vi "Begin.vi"(8 "error in":errorcluster) -> (0 "error out":errorcluster)   [LabVIEW 2018]
doc: "Called before other user functions, this VI is expected to open initial I/O refnums, load in file data, and do all program initialization. Notice that the <B>error out</B> terminal is simply used for data flow. Wiring it to other structures or subVIs ensures that this VI runs first."
uses:
  <vilib>/Rock Robotics/WPI/ThirdParty/Phoenix-LabVIEW/Motor Controller/Controls/CTRE_Phoenix_MotorControl_EnhancedMotorControllerConfigurables.ctl
  <vilib>/Rock Robotics/WPI/ThirdParty/Phoenix-LabVIEW/Motor Controller/Controls/CTRE_Phoenix_MotorControl_BaseConfigurables.ctl
  <vilib>/Rock Robotics/WPI/ThirdParty/Phoenix-LabVIEW/Motor Controller/Controls/CTRE_Phoenix_MotorControl_VelocityMeasurementPeriod.ctl
  <vilib>/Rock Robotics/WPI/ThirdParty/Phoenix-LabVIEW/Motor Controller/Controls/CTRE_Phoenix_MotorControl_SlotStructure.ctl
  <vilib>/Rock Robotics/WPI/ThirdParty/Phoenix-LabVIEW/Motor Controller/Controls/CTRE_Phoenix_MotorControl_FilterStruct.ctl
  <vilib>/Rock Robotics/WPI/ThirdParty/Phoenix-LabVIEW/Motor Controller/Controls/CTRE_Phoenix_MotorControl_RemoteSourceType.ctl
  <vilib>/Rock Robotics/WPI/ThirdParty/Phoenix-LabVIEW/Controls/CTRE_Phoenix_CustomParamConfiguration.ctl
  <vilib>/Rock Robotics/WPI/ThirdParty/Phoenix-LabVIEW/Motor Controller/Controls/CTRE_Phoenix_MotorControl_FeedbackDevice.ctl
  <vilib>/Rock Robotics/WPI/ThirdParty/Phoenix-LabVIEW/Motor Controller/Controls/CTRE_Phoenix_MotorControl_SensorTermFeedbackDevice_Enhanced.ctl
  <vilib>/Rock Robotics/WPI/ThirdParty/Phoenix-LabVIEW/Motor Controller/Controls/CTRE_Phoenix_MotorControl_LimitSwitchNormal.ctl
  <vilib>/Rock Robotics/WPI/ThirdParty/Phoenix-LabVIEW/Motor Controller/Controls/CTRE_Phoenix_MotorControl_LimitSwitchSource_Local.ctl
  <vilib>/Rock Robotics/WPI/ThirdParty/Phoenix-LabVIEW/Motor Controller/Controls/CTRE_Phoenix_MotorControl_MotorControllerConfigurables.ctl
  <vilib>/Rock Robotics/WPI/ThirdParty/Phoenix-LabVIEW/Motor Controller/Controls/CTRE_Phoenix_MotorControl_RemoteFeedbackDevice.ctl
  <vilib>/Rock Robotics/WPI/ThirdParty/Phoenix-LabVIEW/Motor Controller/Controls/CTRE_Phoenix_MotorControl_SensorTermFeedbackDevice.ctl
  <vilib>/Rock Robotics/WPI/ThirdParty/Phoenix-LabVIEW/Motor Controller/Controls/CTRE_Phoenix_MotorControl_LimitSwitchSource.ctl
  <vilib>/Rock Robotics/WPI/DriverStation/WPI_DriverStationRobotMode2.ctl
  <vilib>/Rock Robotics/WPI/Joystick/WPI_JoystickDeviceEnum.ctl
  <vilib>/Rock Robotics/WPI/Solenoid/WPI_SolenoidChannel.ctl
  <vilib>/Rock Robotics/SystemInterfaces/AI/FPGA_AIChannel.ctl
  <vilib>/Rock Robotics/WPI/ThirdParty/Phoenix-LabVIEW/Motor Controller/Controls/CTRE_Phoenix_MotorControl_NeutralMode.ctl
  <vilib>/Rock Robotics/WPI/Accelerometer/WPI_AccelerometerRange.ctl
  <vilib>/Rock Robotics/WPI/ThirdParty/REV Robotics/SPARK MAX/Typedef/Spark MAX Idle Mode.ctl
  <vilib>/Rock Robotics/SystemInterfaces/DIO/FPGA_DIOPWMChannel.ctl
  Robot Global Data.vi
  RefNums_DriverStation.vi
  <vilib>/Rock Robotics/Network Tables/NT Write String Array.vi
  <vilib>/Rock Robotics/WPI/Solenoid/WPI_SolenoidOpenDouble.vi
  RefNums_Actuators.vi
  <vilib>/Rock Robotics/WPI/Utilities/WPI_GetSetVariantRefNum.vi
  RefNums_Sensors.vi
  <vilib>/Rock Robotics/WPI/Accelerometer/InternalAccelerometer/WPI_AccelerometerInternalOpen.vi
  <vilib>/Rock Robotics/WPI/Solenoid/WPI_SolenoidOpenSingle.vi
  <vilib>/Rock Robotics/WPI/SafetyOutput/WPI_SafetyOutputConfigMenu.ctl
  <vilib>/Rock Robotics/WPI/RobotDrive/WPI_RobotDriveOpen4MotorWithExistingMotors.vi
panel:
  in  "Victor Enhanced Control":T1={"Base Configurables"={"openLoopRamp"=0.0, "closedLoopRamp"=0.0, "peakOutputForward"=1.0, "peakOutputReverse"=-1.0, "nominalOutputForward"=0.0, "nominalOutputReverse"=0.0, "neutralDeadband"=0.04, "voltageCompSaturation"=0.0, "voltageMeasurementFilter"=32, "velocityMeasurementPeriod"=100, "velocityMeasurementWindow"=64, "forwardSoftLimitThreshold"=0, "reverseSoftLimitThreshold"=0, "forwardSoftLimitEnable"=FALSE, "reverseSoftLimitEnable"=FALSE, "slot0"={"P"=0.0, "I"=0.0, "D"=0.0, "F"=0.0, "integralZone"=0.0, "allowableClosedLoopError"=0, "maxIntegralAccumulator"=0.0, "closedLoopPeakOutput"=1.0, "closedLoopPeriod"=1}, "slot1"={"P"=0.0, "I"=0.0, "D"=0.0, "F"=0.0, "integralZone"=0.0, "allowableClosedLoopError"=0, "maxIntegralAccumulator"=0.0, "closedLoopPeakOutput"=1.0, "closedLoopPeriod"=1}, "slot2"={"P"=0.0, "I"=0.0, "D"=0.0, "F"=0.0, "integralZone"=0.0, "allowableClosedLoopError"=0, "maxIntegralAccumulator"=0.0, "closedLoopPeakOutput"=1.0, "closedLoopPeriod"=1}, "slot3"={"P"=0.0, "I"=0.0, "D"=0.0, "F"=0.0, "integralZone"=0.0, "allowableClosedLoopError"=0, "maxIntegralAccumulator"=0.0, "closedLoopPeakOutput"=1.0, "closedLoopPeriod"=1}, "auxPIDPolarity"=FALSE, "remoteFilter0"={"remoteSensorDeviceID"=0, "remoteSensorSource"=enum."Off"}, "remoteFilter1"={"remoteSensorDeviceID"=0, "remoteSensorSource"=enum."Off"}, "motionCruiseVelocity"=0, "motionAcceleration"=0, "motionProfileTrajectoryPeriod"=0, "feedbackNotContinuous"=FALSE, "remoteSensorClosedLoopDisableNeutralOnLOS"=FALSE, "clearPositionOnLimitF"=FALSE, "clearPositionOnLimitR"=FALSE, "clearPositionOnQuadIdx"=FALSE, "limitSwitchDisableNeutralOnLOS"=FALSE, "softLimitDisableNeutralOnLOS"=FALSE, "pulseWidthPeriod_EdgesPerRot"=1, "pulseWidthPeriod_FilterWindowSz"=1, "customParam"={"customParam0"=0, "customParam1"=0}, "trajectoryInterpolationEnable"=TRUE}, "primaryPID"={"selectedFeedbackCoefficient"=1.0, "selectedFeedbackSensor"=11}, "auxiliaryPID"={"selectedFeedbackCoefficient"=1.0, "selectedFeedbackSensor"=11}, "sum 0 term"=11, "sum 1 term"=11, "diff 0 term "=11, "diff 1 term"=11, "forwardLimitSwitchDeviceID"=0, "reverseLimitSwitchDeviceID"=0, "forwardLimitSwitchNormal"=enum."Normally Open", "reverseLimitSwitchNormal"=enum."Normally Open", "forwardLimitSwitchSource"=3, "reverseLimitSwitchSource"=3} {"diff 1 term" items=["Remote Source 0"=11, "Remote Source 1"=12, "Software Emulated"=15]; "diff 0 term" items=["Remote Source 0"=11, "Remote Source 1"=12, "Software Emulated"=15]; "sum 1 term" items=["Remote Source 0"=11, "Remote Source 1"=12, "Software Emulated"=15]; "sum 0 term" items=["Remote Source 0"=11, "Remote Source 1"=12, "Software Emulated"=15]; "reverseLimitSwitchSource" items=["Remote Talon SRX"=1, "Remote CANifier"=2, "Deactivated"=3]; "forwardLimitSwitchSource" items=["Remote Talon SRX"=1, "Remote CANifier"=2, "Deactivated"=3]; "auxiliaryPID"."selectedFeedbackSensor" items=["Sensor Sum (S0 + S1)"=9, "Sensor Difference (D0 - D1)"=10, "Remote Source 0"=11, "Remote Source 1"=12, "Software Emulated"=15]; "primaryPID"."selectedFeedbackSensor" items=["Sensor Sum (S0 + S1)"=9, "Sensor Difference (D0 - D1)"=10, "Remote Source 0"=11, "Remote Source 1"=12, "Software Emulated"=15]; "Base Configurables"."velocityMeasurementPeriod" items=["Period_1ms"=1, "Period_2ms"=2, "Period_5ms"=5, "Period_10ms"=10, "Period_20ms"=20, "Period_25ms"=25, "Period_50ms"=50, "Period_100ms"=100]}
  in  "Talon Enhanced Config":T12={"Base Configurables"={"openLoopRamp"=0.0, "closedLoopRamp"=0.0, "peakOutputForward"=1.0, "peakOutputReverse"=-1.0, "nominalOutputForward"=0.0, "nominalOutputReverse"=0.0, "neutralDeadband"=0.04, "voltageCompSaturation"=0.0, "voltageMeasurementFilter"=32, "velocityMeasurementPeriod"=100, "velocityMeasurementWindow"=64, "forwardSoftLimitThreshold"=0, "reverseSoftLimitThreshold"=0, "forwardSoftLimitEnable"=FALSE, "reverseSoftLimitEnable"=FALSE, "slot0"={"P"=0.0, "I"=0.0, "D"=0.0, "F"=0.0, "integralZone"=0.0, "allowableClosedLoopError"=0, "maxIntegralAccumulator"=0.0, "closedLoopPeakOutput"=1.0, "closedLoopPeriod"=1}, "slot1"={"P"=0.0, "I"=0.0, "D"=0.0, "F"=0.0, "integralZone"=0.0, "allowableClosedLoopError"=0, "maxIntegralAccumulator"=0.0, "closedLoopPeakOutput"=1.0, "closedLoopPeriod"=1}, "slot2"={"P"=0.0, "I"=0.0, "D"=0.0, "F"=0.0, "integralZone"=0.0, "allowableClosedLoopError"=0, "maxIntegralAccumulator"=0.0, "closedLoopPeakOutput"=1.0, "closedLoopPeriod"=1}, "slot3"={"P"=0.0, "I"=0.0, "D"=0.0, "F"=0.0, "integralZone"=0.0, "allowableClosedLoopError"=0, "maxIntegralAccumulator"=0.0, "closedLoopPeakOutput"=1.0, "closedLoopPeriod"=1}, "auxPIDPolarity"=FALSE, "remoteFilter0"={"remoteSensorDeviceID"=0, "remoteSensorSource"=enum."Off"}, "remoteFilter1"={"remoteSensorDeviceID"=0, "remoteSensorSource"=enum."Off"}, "motionCruiseVelocity"=0, "motionAcceleration"=0, "motionProfileTrajectoryPeriod"=0, "feedbackNotContinuous"=FALSE, "remoteSensorClosedLoopDisableNeutralOnLOS"=FALSE, "clearPositionOnLimitF"=FALSE, "clearPositionOnLimitR"=FALSE, "clearPositionOnQuadIdx"=FALSE, "limitSwitchDisableNeutralOnLOS"=FALSE, "softLimitDisableNeutralOnLOS"=FALSE, "pulseWidthPeriod_EdgesPerRot"=1, "pulseWidthPeriod_FilterWindowSz"=1, "customParam"={"customParam0"=0, "customParam1"=0}, "trajectoryInterpolationEnable"=TRUE}, "primaryPID"={"selectedFeedbackCoefficient"=1.0, "selectedFeedbackSensor"=0}, "auxiliaryPID"={"selectedFeedbackCoefficient"=1.0, "selectedFeedbackSensor"=0}, "sum0Term"=0, "sum1Term"=0, "diff0Term"=0, "diff1Term"=0, "forwardLimitSwitchNormal"=enum."Normally Open", "reverseLimitSwitchNormal"=enum."Normally Open", "forwardLimitSwitchDeviceID"=0, "reverseLimitSwitchDeviceID"=0, "forwardLimitSwitchSource"=enum."Feedback Connector", "reverseLimitSwitchSource"=enum."Feedback Connector", "peakCurrentLimit"=1, "peakCurrentDuration"=1, "continuousCurrentLimit"=1} {"diff1Term" items=["QuadEncoder"=0, "Analog"=2, "Tachometer"=4, "Pulse Width Encoded Position"=8, "Remote Source 0"=11, "Remote Source 1"=12, "Software Emulated"=15]; "diff0Term" items=["QuadEncoder"=0, "Analog"=2, "Tachometer"=4, "Pulse Width Encoded Position"=8, "Remote Source 0"=11, "Remote Source 1"=12, "Software Emulated"=15]; "sum1Term" items=["QuadEncoder"=0, "Analog"=2, "Tachometer"=4, "Pulse Width Encoded Position"=8, "Remote Source 0"=11, "Remote Source 1"=12, "Software Emulated"=15]; "sum0Term" items=["QuadEncoder"=0, "Analog"=2, "Tachometer"=4, "Pulse Width Encoded Position"=8, "Remote Source 0"=11, "Remote Source 1"=12, "Software Emulated"=15]; "auxiliaryPID"."selectedFeedbackSensor" items=["QuadEncoder"=0, "Analog"=2, "Tachometer"=4, "Pulse Width Encoded Position"=8, "Sensor Sum (S0 + S1)"=9, "Sensor Difference (D0 - D1)"=10, "Remote Source 0"=11, "Remote Source 1"=12, "Software Emulated"=15]; "primaryPID"."selectedFeedbackSensor" items=["QuadEncoder"=0, "Analog"=2, "Tachometer"=4, "Pulse Width Encoded Position"=8, "Sensor Sum (S0 + S1)"=9, "Sensor Difference (D0 - D1)"=10, "Remote Source 0"=11, "Remote Source 1"=12, "Software Emulated"=15]; "Base Configurables"."velocityMeasurementPeriod" items=["Period_1ms"=1, "Period_2ms"=2, "Period_5ms"=5, "Period_10ms"=10, "Period_20ms"=20, "Period_25ms"=25, "Period_50ms"=50, "Period_100ms"=100]}
  # "Sum and Diff terms are ways to select more than one sensor as a feedback device. \n Sum 0 is the first feedback device to be used for the Sum term, \n Sum 1 is the feedback device to be added to Sum 0 for the Sum term\n Diff 0 and Diff 1 work in a similar manner"
  # "These are only applicable\nif using a remote limit switch.\n\nLocal limit switches/no limit\nswitches do not use this"
  # "False: Primary Output = PID[0] + PID[1]  ---  Auxiliary Output = PID[0] - PID[1]\nTrue:  Primary Output = PID[0] - PID[1] --- Auxiliary Output = PID[0] + PID[1]"
  # "Enable the motion profile executor to perform linear interpolation between profile points.  Defaults to True."
  # "Sum and Diff terms are ways to select more than one sensor as a feedback device. \n Sum 0 is the first feedback device to be used for the Sum term.\n Sum 1 is the feedback device to be added to Sum 0 for the Sum term.\n Diff 0 and Diff 1 work in a similar manner."
  # "These are only applicable\nif using a remote limit switch.\n\nLocal limit switches/no limit\nswitches do not use this."
  # "Current is below Continuous threshold AND\n\n(Requested output is weaker** than applied motor\noutput OR is in the opposite direction).\n/\nMotor output is set to requested output."
  # "Current is above Peak* Threshold for Peak Duration.\n/\nReduce motor output (towards neutral)."
  # "Current is below Continuous threshold.\n/\nRamp motor output towards requested output."
  # "Current is above Continuous threshold.\n/\nReduce motor output (towards neutral)."
  # "Current Limiting is NOT enabled\nby default.\nCall this VI to enable."
  # "*If the configured Peak Threshold is less than the Continuous Threshold, the applied Peak Threshold is set equal to the Configured Continuous Threshold in firmware.\n** Both requested output and applied motor output are in the same direction, and requested output is closer to neutral."
  # "False: Primary Output = PID[0] + PID[1]  ---  Auxiliary Output = PID[0] - PID[1]\nTrue:  Primary Output = PID[0] - PID[1] --- Auxiliary Output = PID[0] + PID[1]"
  # "Enable the motion profile executor to perform linear interpolation between profile points.  Defaults to True."
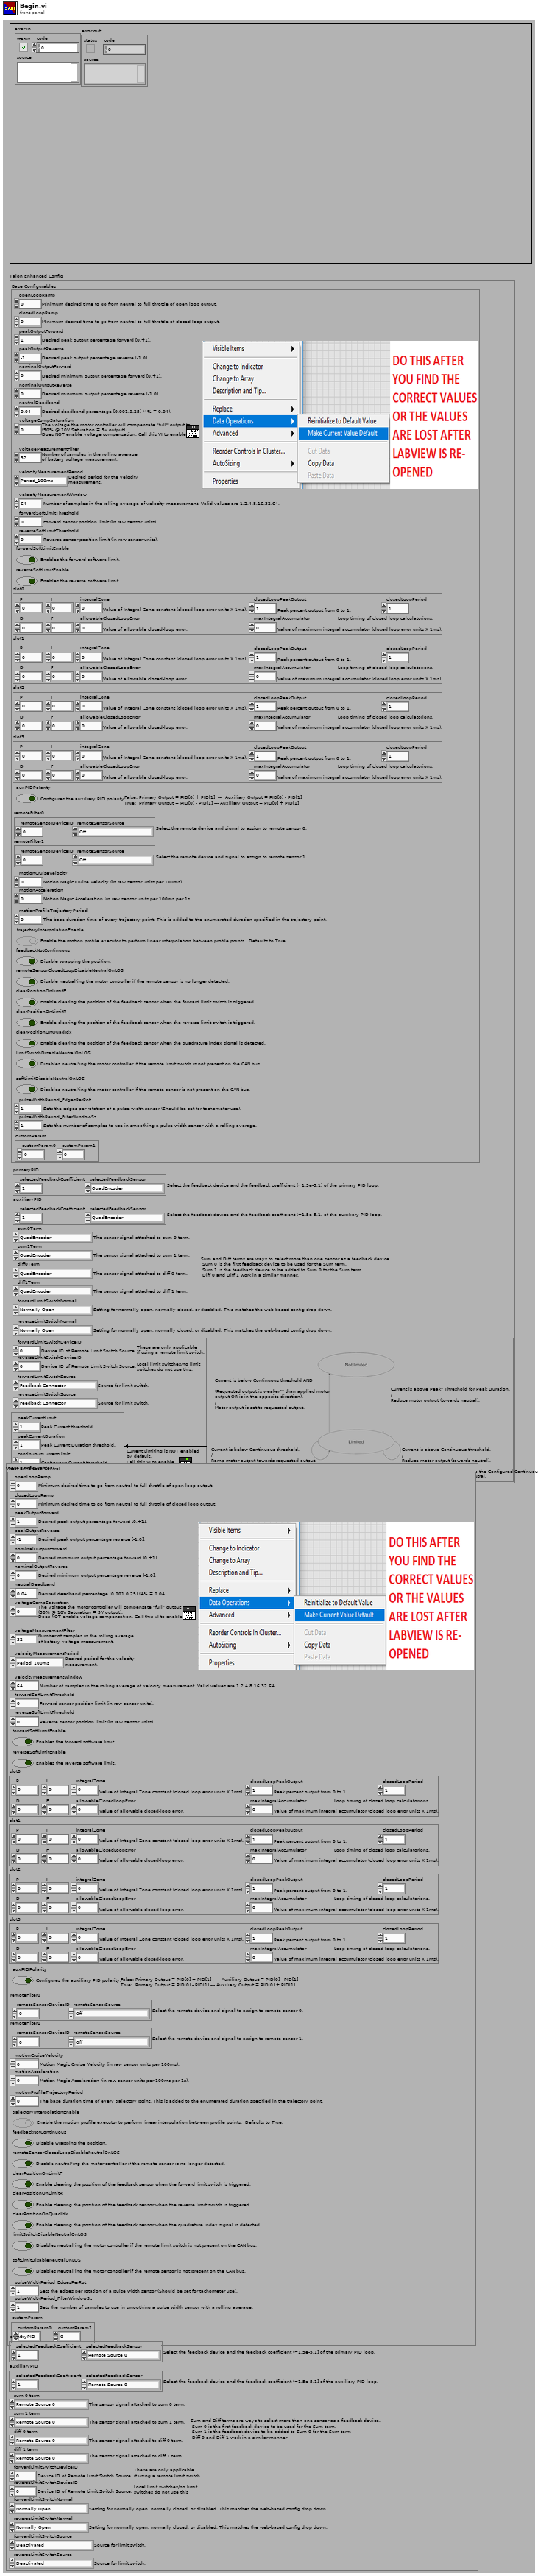
[diagram p1: front panel]
types:
  T1 = typedef "CTRE_Phoenix_MotorControl_MotorControllerConfigurables.ctl" = cluster{"Base Configurables":T2, "primaryPID":cluster{"selectedFeedbackCoefficient":dbl, "selectedFeedbackSensor":T8}, "auxiliaryPID":cluster{"selectedFeedbackCoefficient":dbl, "selectedFeedbackSensor":T8}, "sum 0 term":T9, "sum 1 term":T9, "diff 0 term ":T9, "diff 1 term":T9, "forwardLimitSwitchDeviceID":i32, "reverseLimitSwitchDeviceID":i32, "forwardLimitSwitchNormal":T10, "reverseLimitSwitchNormal":T10, "forwardLimitSwitchSource":T11, "reverseLimitSwitchSource":T11}
  T2 = typedef "CTRE_Phoenix_MotorControl_BaseConfigurables.ctl" = cluster{"openLoopRamp":dbl, "closedLoopRamp":dbl, "peakOutputForward":dbl, "peakOutputReverse":dbl, "nominalOutputForward":dbl, "nominalOutputReverse":dbl, "neutralDeadband":dbl, "voltageCompSaturation":dbl, "voltageMeasurementFilter":i32, "velocityMeasurementPeriod":T3, "velocityMeasurementWindow":i32, "forwardSoftLimitThreshold":i32, "reverseSoftLimitThreshold":i32, "forwardSoftLimitEnable":bool, "reverseSoftLimitEnable":bool, "slot0":T4, "slot1":T4, "slot2":T4, "slot3":T4, "auxPIDPolarity":bool, "remoteFilter0":T5, "remoteFilter1":T5, "motionCruiseVelocity":i32, "motionAcceleration":i32, "motionProfileTrajectoryPeriod":i32, "feedbackNotContinuous":bool, "remoteSensorClosedLoopDisableNeutralOnLOS":bool, "clearPositionOnLimitF":bool, "clearPositionOnLimitR":bool, "clearPositionOnQuadIdx":bool, "limitSwitchDisableNeutralOnLOS":bool, "softLimitDisableNeutralOnLOS":bool, "pulseWidthPeriod_EdgesPerRot":i32, "pulseWidthPeriod_FilterWindowSz":i32, "customParam":T7, "trajectoryInterpolationEnable":bool}
  T3 = typedef "CTRE_Phoenix_MotorControl_VelocityMeasurementPeriod.ctl" = u16
  T4 = typedef "CTRE_Phoenix_MotorControl_SlotStructure.ctl" = cluster{"P":dbl, "I":dbl, "D":dbl, "F":dbl, "integralZone":dbl, "allowableClosedLoopError":i32, "maxIntegralAccumulator":dbl, "closedLoopPeakOutput":dbl, "closedLoopPeriod":i32}
  T5 = typedef "CTRE_Phoenix_MotorControl_FilterStruct.ctl" = cluster{"remoteSensorDeviceID":u8, "remoteSensorSource":T6}
  T6 = typedef "CTRE_Phoenix_MotorControl_RemoteSourceType.ctl" = enum16{"Off", "Talon SRX Selected Sensor", "Pigeon IMU Yaw", "Pigeon IMU Pitch", "Pigeon IMU Roll", "CANifier Quadrature", "CANifier PWM Input 0", "CANifier PWM Input 1", "CANifier PWM Input 2", "CANifier PWM Input 3", "Gadgeteer Pigeon Yaw", "Gadgeteer Pigeon Pitch", "Gadgeteer Pigeon Roll"}
  T7 = typedef "CTRE_Phoenix_CustomParamConfiguration.ctl" = cluster{"customParam0":i32, "customParam1":i32}
  T8 = typedef "CTRE_Phoenix_MotorControl_RemoteFeedbackDevice.ctl" = i8
  T9 = typedef "CTRE_Phoenix_MotorControl_SensorTermFeedbackDevice.ctl" = i8
  T10 = typedef "CTRE_Phoenix_MotorControl_LimitSwitchNormal.ctl" = enum16{"Normally Open", "Normally Closed", "Disabled"}
  T11 = typedef "CTRE_Phoenix_MotorControl_LimitSwitchSource.ctl" = u16
  T12 = typedef "CTRE_Phoenix_MotorControl_EnhancedMotorControllerConfigurables.ctl" = cluster{"Base Configurables":T2, "primaryPID":cluster{"selectedFeedbackCoefficient":dbl, "selectedFeedbackSensor":T13}, "auxiliaryPID":cluster{"selectedFeedbackCoefficient":dbl, "selectedFeedbackSensor":T13}, "sum0Term":T14, "sum1Term":T14, "diff0Term":T14, "diff1Term":T14, "forwardLimitSwitchNormal":T10, "reverseLimitSwitchNormal":T10, "forwardLimitSwitchDeviceID":i32, "reverseLimitSwitchDeviceID":i32, "forwardLimitSwitchSource":T15, "reverseLimitSwitchSource":T15, "peakCurrentLimit":i32, "peakCurrentDuration":i32, "continuousCurrentLimit":i32}
  T13 = typedef "CTRE_Phoenix_MotorControl_FeedbackDevice.ctl" = i8
  T14 = typedef "CTRE_Phoenix_MotorControl_SensorTermFeedbackDevice_Enhanced.ctl" = i8
  T15 = typedef "CTRE_Phoenix_MotorControl_LimitSwitchSource_Local.ctl" = enum16{"Feedback Connector", "Remote Talon SRX", "Remote CANifier", "Deactivated"}
  T16 = typedef "FPGA_DIOPWMChannel.ctl" = enum8{"PWM 0", "PWM 1", "PWM 2", "PWM 3", "PWM 4", "PWM 5", "PWM 6", "PWM 7", "PWM 8", "PWM 9", "PWM MXP 0", "PWM MXP 1", "PWM MXP 2", "PWM MXP 3", "PWM MXP 4", "PWM MXP 5", "PWM MXP 6", "PWM MXP 7", "PWM MXP 8", "PWM MXP 9", "Invalid"}
  T17 = typedef "Spark MAX Idle Mode.ctl" = enum16{"Coast", "Brake"}
  T18 = typedef "WPI_SolenoidChannel.ctl" = enum8{"Solenoid 0", "Solenoid 1", "Solenoid 2", "Solenoid 3", "Solenoid 4", "Solenoid 5", "Solenoid 6", "Solenoid 7", "Invalid"}
  T19 = typedef "WPI_AccelerometerRange.ctl" = enum16{"+/- 2 g", "+/- 4 g", "+/- 8 g"}
  T20 = typedef "WPI_JoystickDeviceEnum.ctl" = enum16{"USB 0", "USB 1", "USB 2", "USB 3", "USB 4", "USB 5"}
  T21 = typedef "CTRE_Phoenix_MotorControl_NeutralMode.ctl" = enum8{"EEPROMSetting", "Override to Coast", "Override to Brake"}
  T22 = typedef "FPGA_AIChannel.ctl" = enum8{"AI 0", "AI 1", "AI 2", "AI 3", "AI MXP 0", "AI MXP 1", "AI MXP 2", "AI MXP 3", "Invalid"}
  T23 = typedef "WPI_DriverStationRobotMode2.ctl" = enum16{"Autonomous Disabled", "Autonomous Enabled", "Teleop Disabled", "Teleop Enabled", "Disconnected", "Finish", "Test Disabled", "Test Enabled", "Emergency Stopped"}
  T24 = typedef "WPI_JoystickDevRef.ctl" = cluster{"Device":T20}
  T25 = typedef "WPI_SolenoidDevRef.ctl" = cluster{"DevStatus":errorcluster, "Pneumatics Control Module":u8, "Forward Solenoid Channel":T18, "Reverse Solenoid Channel":T18}
  T26 = typedef "WPI_CompressorDevRef.ctl" = cluster{"DevStatus":errorcluster, "Pneumatics Control Module":u8}
  T27 = typedef "WPI_MotorControlDeviceRef.ctl" = cluster{"DeviceStatus":errorcluster, "Type":T28, "PWM":cluster{"PWM Channel":T16, "DeadBand":T29}, "CAN":cluster{"Device Number":u8, "SetOutput VI Ref":variant, "GetOutput VI Ref":variant, "Enable VI Ref":variant, "Disable VI Ref":variant, "Data":variant}, "Invert":bool, "DIO PWM":cluster{"PWM \"Enable\" Channel":T16, "DIOChannel":T30, "PWM Rate":dbl}}
  T28 = typedef "WPI_MotorControlType.ctl" = enum16{"PWM", "CAN", "DIO PWM"}
  T29 = typedef "WPI_PWMDeadband.ctl" = cluster{"Name":string, "maxPositivePwm":i32, "minPositivePwm":i32, "centerPwm":i32, "maxNegativePwm":i32, "minNegativePwm":i32, "angularRange":u16}
  T30 = typedef "FPGA_DIOChannel.ctl" = enum8{"DIO 0", "DIO 1", "DIO 2", "DIO 3", "DIO 4", "DIO 5", "DIO 6", "DIO 7", "DIO 8", "DIO 9", "DIO MXP 0", "DIO MXP 1", "DIO MXP 2", "DIO MXP 3", "DIO MXP 4", "DIO MXP 5", "DIO MXP 6", "DIO MXP 7", "DIO MXP 8", "DIO MXP 9", "DIO MXP 10", "DIO MXP 11", "DIO MXP 12", "DIO MXP 13", "DIO MXP 14", "DIO MXP 15", "SPI Port CS1", "SPI Port CS2", "SPI Port CS3", "SPI Port MISO", "SPI Port MOSI", "Invalid"}
  T31 = typedef "WPI_SafetyOutputConfigMenu.ctl" = enum16{"Enable", "Disable"}
  T32 = typedef "WPI_RobotDriveDevRef.ctl" = cluster{"DevStatus":errorcluster, "Motors[]":T27[], "Square Inputs":bool, "Max Output":dbl}
  T33 = typedef "WPI_ServoDeviceRef.ctl" = cluster{"DeviceStatus":errorcluster, "PWM Channel":T16, "DeadBand":T29}
  T34 = typedef "WPI_AnalogChannelDevRef.ctl" = cluster{"DevStatus":errorcluster, "Analog Channel":T22}
  T35 = typedef "WPI_AccelerometerDevRef.ctl" = cluster{"DevStatus":errorcluster, "Scaling":T36, "Analog Channels":T37, "I2C Bus":T38, "SPI Bus":T39, "Accel Range":T40, "ADXL Axes":T41, "Handle":i32, "Device Address":u8, "Accel Type":enum16{"Analog", "ADXL345 I2C", "ADXL345 SPI", "Internal", "ADXL362 SPI"}}
  T36 = typedef "WPI_AccelerometerScaling.ctl" = cluster{"Gain (VoltsPerG)":dbl, "Center Voltage":dbl}
  T37 = typedef "WPI_AccelerometerAnalogChannels.ctl" = cluster{"X-Axis":T22, "Y-Axis":T22, "Z-Axis":T22}
  T38 = typedef "i2c_bus.ctl" = enum16{"I2C On-Board", "I2C MXP", "Invalid"}
  T39 = typedef "spi_bus.ctl" = enum16{"SPI On-Board, CS0", "SPI On-Board, CS1", "SPI On-Board, CS2", "SPI On-Board, CS3", "SPI MXP", "Invalid"}
  T40 = typedef "ADXL345 Range.ctl" = u8
  T41 = typedef "WPI_AccelerometerADXL345 Axes.ctl" = cluster{"X-Axis":bool, "Y-Axis":bool, "Z-Axis":bool}
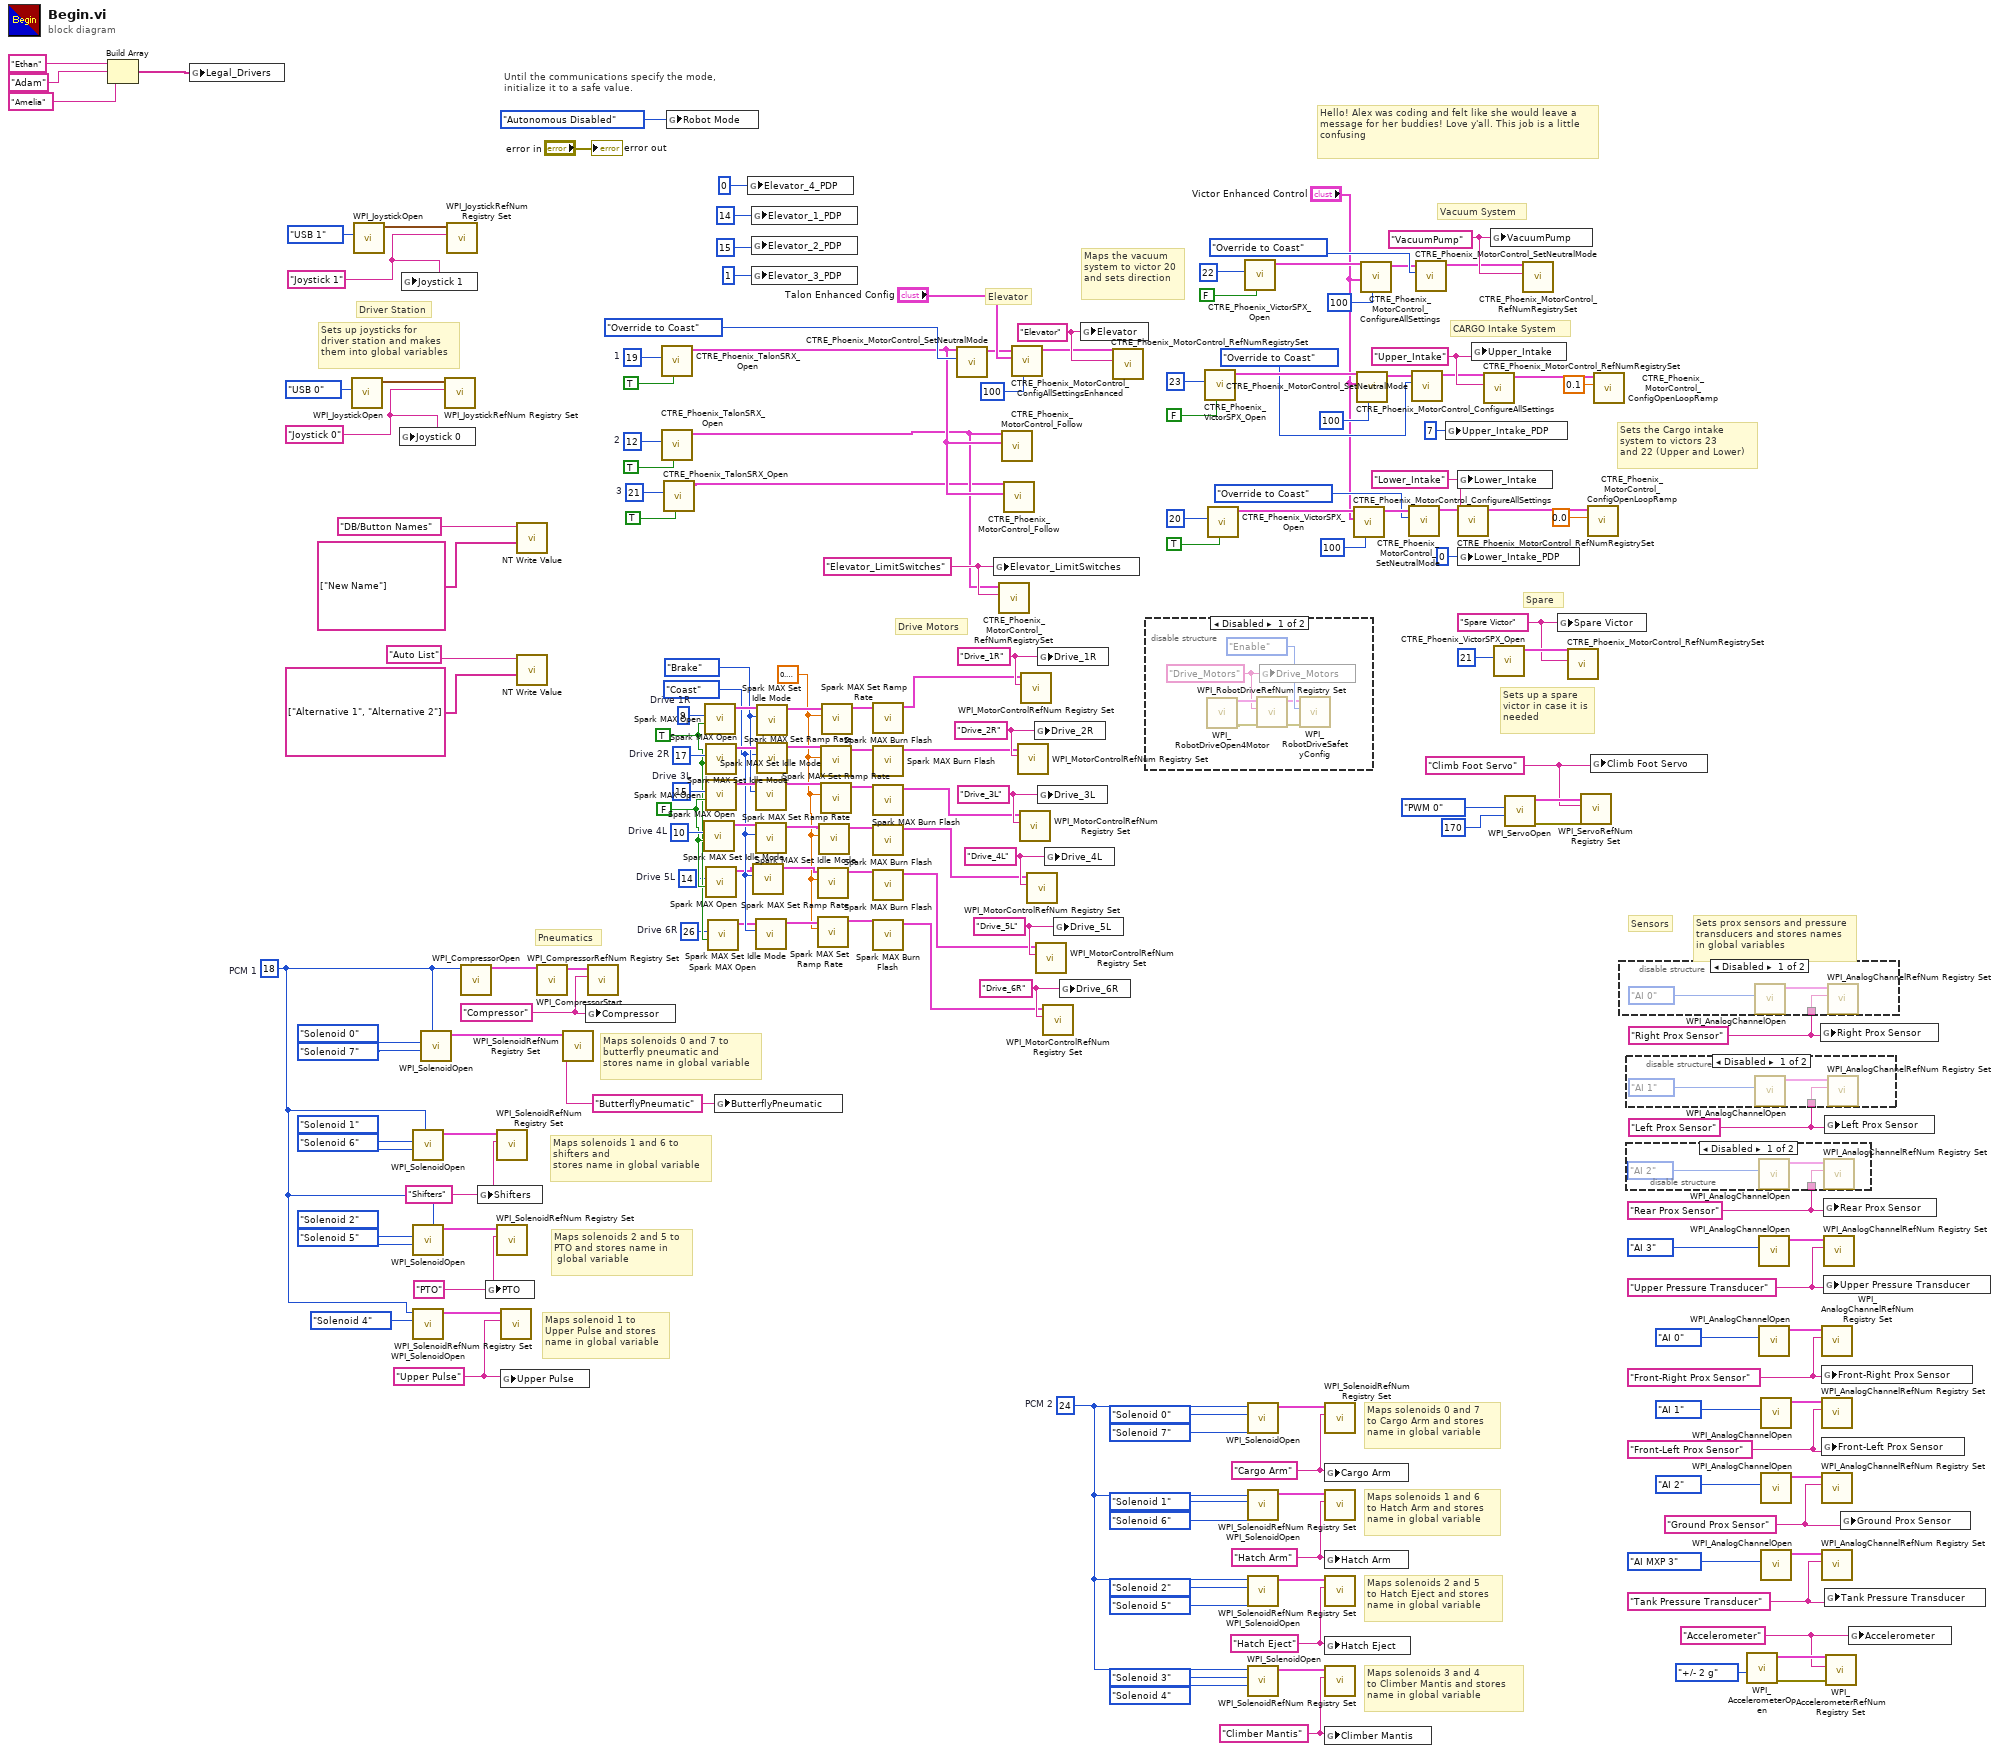
[diagram p0: block diagram]
diagram:
  w21 = u8 26  # Drive 6R
  w22 = u8 14  # Drive 5L
  w31 = "Drive_6R" ("refnum name")
  w32 = "Drive_5L" ("refnum name")
  w33 = "Climb Foot Servo" ("refnum name")
  w23 = sgl 0.1 ("Seconds from neutral to full (0)")
  w30 = Spark_MAX_Idle_Mode."Coast" ("Idle Mode")
  w50 = u8 21  # 3
  w52 = "Upper Pulse" ("ButterflyPneumatic")
  w46 = Spark_MAX_Idle_Mode."Brake" ("Idle Mode")
  w57 = "Accelerometer" ("refnum name")
  w61 = "Drive_4L" ("refnum name")
  w62 = "Drive_3L" ("refnum name")
  w63 = "Drive_2R" ("refnum name")
  w64 = "Drive_1R" ("refnum name")
  w65 = "Elevator_LimitSwitches" ("refnum name")
  w29 = FALSE ("Invert")
  w66 = u8 10  # Drive 4L
  w67 = u8 15  # Drive 3L
  w68 = u8 17  # Drive 2R
  w28 = TRUE ("Invert")
  w69 = u8 9  # Drive 1R
  w71 = "Joystick 1" ("refnum name")
  w90 = u8 12  # 2
  w95 = "Tank Pressure Transducer" ("refnum name")
  w98 = "Ground Prox Sensor" ("refnum name")
  w101 = "Front-Left Prox Sensor" ("refnum name")
  w104 = "Front-Right Prox Sensor" ("refnum name")
  w108 = "Climber Mantis" ("ButterflyPneumatic")
  w112 = "Hatch Eject" ("ButterflyPneumatic")
  w116 = "Hatch Arm" ("ButterflyPneumatic")
  w107 = u8 24  # PCM 2
  w120 = "PTO" ("ButterflyPneumatic")
  w124 = "Spare Victor" ("refnum name")
  w127 = "Upper Pressure Transducer" ("refnum name")
  w130 = "Rear Prox Sensor" ("refnum name")
  w131 = "Left Prox Sensor" ("refnum name")
  w132 = "Right Prox Sensor" ("refnum name")
  w133 = "Elevator" ("refnum name")
  w135 = u8 19  # 1
  w141 = "Lower_Intake" ("refnum name")
  w142 = "Upper_Intake" ("refnum name")
  w147 = "Cargo Arm" ("ButterflyPneumatic")
  w151 = "VacuumPump" ("refnum name")
  w154 = "Shifters" ("ButterflyPneumatic")
  w158 = "Compressor" ("Compressor")
  w159 = "ButterflyPneumatic" ("ButterflyPneumatic")
  w51 = u8 18  # PCM 1
  w165 = "Joystick 0" ("refnum name")
  # "Hello! Alex was coding and felt like she would leave a message for her buddies! Love y'all. This job is a little confusing"
  # "Maps solenoid 1 to\nUpper Pulse and stores \nname in global variable"
  # "Drive Motors"
  # "Sets the Cargo intake \nsystem to victors 23 \nand 22 (Upper and Lower)"
  # "Maps the vacuum\nsystem to victor 20\nand sets direction"
  # "Sets up a spare\nvictor in case it is\nneeded"
  # "Sets up joysticks for\ndriver station and makes\nthem into global variables"
  # "Maps solenoids 3 and 4\nto Climber Mantis and stores \nname in global variable"
  # "Maps solenoids 2 and 5\nto Hatch Eject and stores \nname in global variable"
  # "Maps solenoids 1 and 6\nto Hatch Arm and stores \nname in global variable"
  # "Maps solenoids 0 and 7\nto Cargo Arm and stores \nname in global variable"
  # "Maps solenoids 2 and 5 to\nPTO and stores name in\n global variable"
  # "Maps solenoids 1 and 6 to\nshifters and \nstores name in global variable"
  # "Maps solenoids 0 and 7 to\nbutterfly pneumatic and \nstores name in global variable"
  # "Sets prox sensors and pressure\ntransducers and stores names \nin global variables"
  # "Spare"
  # "CARGO Intake System"
  # "Vacuum System"
  # "Elevator"
  # "Sensors"
  # "Pneumatics"
  # "Driver Station"
  # "Until the communications specify the mode,\ninitialize it to a safe value."
  n1 = Build Array("Ethan", "Adam" ("element"), "Amelia" ("element")) -> (w1:string[])
  n2 = global write "RefNums_DriverStation.vi" "Legal_Drivers"(w1) -> ()
  n3 = call <vilib>:"WPI_JoystickOpen.vi"("JoystickDevice"=WPI_JoystickDeviceEnum."USB 0") -> ("JoystickDevRef"=w172:T24)  [unwired: 10 in]
  n4 = call <vilib>:"WPI_JoystickOpen.vi"("JoystickDevice"=WPI_JoystickDeviceEnum."USB 1") -> ("JoystickDevRef"=w70:T24)  [unwired: 10 in]
  n5 = global write "RefNums_DriverStation.vi" "Joystick 0"(w165) -> ()
  n6 = global write "RefNums_DriverStation.vi" "Joystick 1"(w71) -> ()
  n7 = call-poly <vilib>:"WPI_SolenoidOpen.vi"("Reverse Solenoid Channel"=WPI_SolenoidChannel."Solenoid 6", "Forward Solenoid Channel"=WPI_SolenoidChannel."Solenoid 1", "Pneumatics Control Module (0)"=w51) -> ("SolenoidDevRef"=w155:T25)  [unwired: 7 in, 1 out]
  n8 = call-poly <vilib>:"WPI_SolenoidOpen.vi"("Reverse Solenoid Channel"=WPI_SolenoidChannel."Solenoid 5", "Forward Solenoid Channel"=WPI_SolenoidChannel."Solenoid 2", "Pneumatics Control Module (0)"=w51) -> ("SolenoidDevRef"=w121:T25)  [unwired: 7 in, 1 out]
  n9 = call-poly <vilib>:"WPI_SolenoidOpen.vi"("Solenoid Channel"=WPI_SolenoidChannel."Solenoid 4" ("Forward Solenoid Channel"), "Pneumatics Control Module (0)"=w51) -> ("SolenoidDevRef"=w53:T25)  [unwired: 8 in, 1 out]
  n10 = call-poly <vilib>:"WPI_SolenoidOpen.vi"("Reverse Solenoid Channel"=WPI_SolenoidChannel."Solenoid 7", "Forward Solenoid Channel"=WPI_SolenoidChannel."Solenoid 0", "Pneumatics Control Module (0)"=w51) -> ("SolenoidDevRef"=w161:T25)  [unwired: 7 in, 1 out]
  n11 = call <vilib>:"WPI_JoystickRefNum Registry Set.vi"("refnum name"=w165, "JoystickDevRef"=w172) -> ()  [unwired: 8 in, 2 out]
  n12 = call <vilib>:"WPI_JoystickRefNum Registry Set.vi"("refnum name"=w71, "JoystickDevRef"=w70) -> ()  [unwired: 8 in, 2 out]
  n13 = call <vilib>:"WPI_CompressorOpen.vi"("Pneumatics Control Module (0)"=w51) -> ("CompressorDevRef"=w164:T26)  [unwired: 13 in, 1 out]
  n14 = global write "RefNums_Actuators.vi" "Shifters"(w154) -> ()
  n15 = global write "RefNums_Actuators.vi" "PTO"(w120) -> ()
  n16 = call <vilib>:"WPI_SolenoidRefNum Registry Set.vi"("refnum name"=w154, "SolenoidDevRef"=w155) -> ()  [unwired: 8 in, 2 out]
  n17 = call <vilib>:"WPI_SolenoidRefNum Registry Set.vi"("refnum name"=w120, "SolenoidDevRef"=w121) -> ()  [unwired: 8 in, 2 out]
  n18 = call <vilib>:"WPI_SolenoidRefNum Registry Set.vi"("refnum name"=w52, "SolenoidDevRef"=w53) -> ()  [unwired: 8 in, 2 out]
  n19 = global write "RefNums_Actuators.vi" "Upper Pulse"(w52) -> ()
  n20 = call-poly <vilib>:"NT Write Value.vi"("String Array"=string[] ["New Name"], "Name"="DB/Button Names") -> ()  [unwired: 9 in, 1 out]
  n21 = call-poly <vilib>:"NT Write Value.vi"("String Array"=string[] ["Alternative 1", "Alternative 2"], "Name"="Auto List") -> ()  [unwired: 9 in, 1 out]
  n22 = call <vilib>:"WPI_CompressorStart.vi"("CompressorDevRef"=w164) -> ("CompressorDevRef"=w160:T26)  [unwired: 9 in, 1 out]
  n23 = call <vilib>:"WPI_SolenoidRefNum Registry Set.vi"("refnum name"=w159, "SolenoidDevRef"=w161) -> ()  [unwired: 8 in, 2 out]
  n24 = global write "RefNums_Actuators.vi" "Compressor"(w158) -> ()
  n25 = call <vilib>:"WPI_CompressorRefNum Registry Set.vi"("refnum name"=w158, "CompressorDevRef"=w160) -> ()  [unwired: 8 in, 2 out]
  n26 = call <vilib>:"CTRE_Phoenix_TalonSRX_Open.vi"("Invert"=TRUE, "Device Number"=w135) -> ("CAN Talon SRX Ref"=w19:T27)  [unwired: 8 in, 1 out]
  n27 = call <vilib>:"CTRE_Phoenix_TalonSRX_Open.vi"("Invert"=TRUE, "Device Number"=w90) -> ("CAN Talon SRX Ref"=w18:T27)  [unwired: 8 in, 1 out]
  n28 = call <vilib>:"CTRE_Phoenix_TalonSRX_Open.vi"("Invert"=TRUE, "Device Number"=w50) -> ("CAN Talon SRX Ref"=w17:T27)  [unwired: 8 in, 1 out]
  n29 = global write "Robot Global Data.vi" "Robot Mode"(WPI_DriverStationRobotMode2."Autonomous Disabled" ("Robot Mode")) -> ()
  n30 = call <vilib>:"Spark MAX Open.vi"("Invert"=w29, "Device Number"=w66) -> ("MotorControlDeviceRef"=w47:T27)  [unwired: 8 in, 1 out]
  n31 = call <vilib>:"Spark MAX Open.vi"("Invert"=w28, "Device Number"=w69) -> ("MotorControlDeviceRef"=w56:T27)  [unwired: 8 in, 1 out]
  n32 = call <vilib>:"Spark MAX Open.vi"("Invert"=w28, "Device Number"=w68) -> ("MotorControlDeviceRef"=w48:T27)  [unwired: 8 in, 1 out]
  n33 = call <vilib>:"Spark MAX Open.vi"("Invert"=w29, "Device Number"=w67) -> ("MotorControlDeviceRef"=w55:T27)  [unwired: 8 in, 1 out]
  n34 = call <vilib>:"Spark MAX Open.vi"("Invert"=w29, "Device Number"=w22) -> ("MotorControlDeviceRef"=w27:T27)  [unwired: 8 in, 1 out]
  n35 = call <vilib>:"Spark MAX Open.vi"("Invert"=w28, "Device Number"=w21) -> ("MotorControlDeviceRef"=w26:T27)  [unwired: 8 in, 1 out]
  n36 = global write "RefNums_Actuators.vi" "ButterflyPneumatic"(w159) -> ()
  n37 = global write "RefNums_Actuators.vi" "Elevator_4_PDP"(0 ("Lower_Intake_PDP")) -> ()
  n38 = global write "RefNums_Actuators.vi" "Elevator_1_PDP"(14 ("Lower_Intake_PDP")) -> ()
  n39 = global write "RefNums_Actuators.vi" "Elevator_2_PDP"(15 ("Lower_Intake_PDP")) -> ()
  n40 = global write "RefNums_Actuators.vi" "Elevator_3_PDP"(1 ("Lower_Intake_PDP")) -> ()
  n41 = call <vilib>:"Spark MAX Set Idle Mode.vi"("Idle Mode"=w30, "MotorControlDeviceRef in"=w27) -> ("MotorControlDeviceRef out"=w25:T27)  [unwired: 8 in, 1 out]
  n42 = call <vilib>:"Spark MAX Set Idle Mode.vi"("Idle Mode"=w46, "MotorControlDeviceRef in"=w55) -> ("MotorControlDeviceRef out"=w43:T27)  [unwired: 8 in, 1 out]
  n43 = call <vilib>:"Spark MAX Set Idle Mode.vi"("Idle Mode"=w30, "MotorControlDeviceRef in"=w47) -> ("MotorControlDeviceRef out"=w44:T27)  [unwired: 8 in, 1 out]
  n44 = call <vilib>:"Spark MAX Set Idle Mode.vi"("Idle Mode"=w30, "MotorControlDeviceRef in"=w26) -> ("MotorControlDeviceRef out"=w24:T27)  [unwired: 8 in, 1 out]
  n45 = call <vilib>:"Spark MAX Set Idle Mode.vi"("Idle Mode"=w46, "MotorControlDeviceRef in"=w56) -> ("MotorControlDeviceRef out"=w45:T27)  [unwired: 8 in, 1 out]
  n46 = call <vilib>:"Spark MAX Set Idle Mode.vi"("Idle Mode"=w30, "MotorControlDeviceRef in"=w48) -> ("MotorControlDeviceRef out"=w42:T27)  [unwired: 8 in, 1 out]
  n47 = call <vilib>:"Spark MAX Set Ramp Rate.vi"("Seconds from neutral to full (0)"=w23, "MotorControlDeviceRef in"=w25) -> ("MotorControlDeviceRef"=w8:T27)  [unwired: 8 in, 1 out]
  n48 = call <vilib>:"Spark MAX Set Ramp Rate.vi"("Seconds from neutral to full (0)"=w23, "MotorControlDeviceRef in"=w24) -> ("MotorControlDeviceRef"=w6:T27)  [unwired: 8 in, 1 out]
  n49 = call <vilib>:"Spark MAX Set Ramp Rate.vi"("Seconds from neutral to full (0)"=w23, "MotorControlDeviceRef in"=w44) -> ("MotorControlDeviceRef"=w10:T27)  [unwired: 8 in, 1 out]
  n50 = call <vilib>:"Spark MAX Set Ramp Rate.vi"("Seconds from neutral to full (0)"=w23, "MotorControlDeviceRef in"=w42) -> ("MotorControlDeviceRef"=w14:T27)  [unwired: 8 in, 1 out]
  n51 = call <vilib>:"Spark MAX Set Ramp Rate.vi"("Seconds from neutral to full (0)"=w23, "MotorControlDeviceRef in"=w43) -> ("MotorControlDeviceRef"=w12:T27)  [unwired: 8 in, 1 out]
  n52 = call <vilib>:"Spark MAX Set Ramp Rate.vi"("Seconds from neutral to full (0)"=w23, "MotorControlDeviceRef in"=w45) -> ("MotorControlDeviceRef"=w16:T27)  [unwired: 8 in, 1 out]
  n53 = call <vilib>:"Spark MAX Burn Flash.vi"("MotorControlDeviceRef"=w16) -> ("MotorControlDeviceRef"=w15:T27)  [unwired: 9 in, 1 out]
  n54 = call <vilib>:"Spark MAX Burn Flash.vi"("MotorControlDeviceRef"=w14) -> ("MotorControlDeviceRef"=w13:T27)  [unwired: 9 in, 1 out]
  n55 = call <vilib>:"Spark MAX Burn Flash.vi"("MotorControlDeviceRef"=w12) -> ("MotorControlDeviceRef"=w11:T27)  [unwired: 9 in, 1 out]
  n56 = call <vilib>:"Spark MAX Burn Flash.vi"("MotorControlDeviceRef"=w10) -> ("MotorControlDeviceRef"=w9:T27)  [unwired: 9 in, 1 out]
  n57 = call <vilib>:"Spark MAX Burn Flash.vi"("MotorControlDeviceRef"=w8) -> ("MotorControlDeviceRef"=w7:T27)  [unwired: 9 in, 1 out]
  n58 = call <vilib>:"Spark MAX Burn Flash.vi"("MotorControlDeviceRef"=w6) -> ("MotorControlDeviceRef"=w5:T27)  [unwired: 9 in, 1 out]
  n59 = call <vilib>:"CTRE_Phoenix_MotorControl_SetNeutralMode.vi"("Motor Control Neutral Mode"=CTRE_Phoenix_MotorControl_NeutralMode."Override to Coast", "PhoenixMotorControlDevRef"=w19) -> ("PhoenixMotorControlDevRef"=w93:T27)  [unwired: 8 in, 1 out]
  n60 = global write "RefNums_Actuators.vi" "Elevator_LimitSwitches"(w65) -> ()
  n61 = call <vilib>:"CTRE_Phoenix_MotorControl_RefNumRegistrySet.vi"("refnum name"=w65, "PhoenixMotorControlDevRef"=w18) -> ()  [unwired: 8 in, 2 out]
  n62 = call <vilib>:"CTRE_Phoenix_MotorControl_Follow.vi"("Master Controller to Follow"=w19, "PhoenixMotorControlDevRef"=w18) -> ()  [unwired: 8 in, 2 out]
  n63 = call <vilib>:"CTRE_Phoenix_MotorControl_Follow.vi"("Master Controller to Follow"=w19, "PhoenixMotorControlDevRef"=w17) -> ()  [unwired: 8 in, 2 out]
  n64 = call <vilib>:"CTRE_Phoenix_MotorControl_ConfigAllSettingsEnhanced.vi"("timeoutMs"=100, "Enhanced Motor Controller Configurables"="Talon Enhanced Config", "PhoenixMotorControlDevRef"=w93) -> ("PhoenixMotorControlDevRef"=w92:T27)  [unwired: 7 in, 1 out]
  n65 = call <vilib>:"WPI_MotorControlRefNum Registry Set.vi"("refnum name"=w63, "MotorControlDevRef"=w13) -> ()  [unwired: 8 in, 2 out]
  n66 = call <vilib>:"WPI_MotorControlRefNum Registry Set.vi"("refnum name"=w62, "MotorControlDevRef"=w11) -> ()  [unwired: 8 in, 2 out]
  n67 = call <vilib>:"WPI_MotorControlRefNum Registry Set.vi"("refnum name"=w64, "MotorControlDevRef"=w15) -> ()  [unwired: 8 in, 2 out]
  n68 = call <vilib>:"WPI_MotorControlRefNum Registry Set.vi"("refnum name"=w61, "MotorControlDevRef"=w9) -> ()  [unwired: 8 in, 2 out]
  n69 = global write "RefNums_Actuators.vi" "Drive_2R"(w63) -> ()
  n70 = call <vilib>:"WPI_MotorControlRefNum Registry Set.vi"("refnum name"=w32, "MotorControlDevRef"=w7) -> ()  [unwired: 8 in, 2 out]
  n71 = global write "RefNums_Actuators.vi" "Drive_1R"(w64) -> ()
  n72 = global write "RefNums_Actuators.vi" "Drive_3L"(w62) -> ()
  n73 = call <vilib>:"WPI_MotorControlRefNum Registry Set.vi"("refnum name"=w31, "MotorControlDevRef"=w5) -> ()  [unwired: 8 in, 2 out]
  n74 = global write "RefNums_Actuators.vi" "Drive_4L"(w61) -> ()
  n75 = global write "RefNums_Actuators.vi" "Drive_5L"(w32) -> ()
  n76 = global write "RefNums_Actuators.vi" "Drive_6R"(w31) -> ()
  n77 = global write "RefNums_Actuators.vi" "Elevator"(w133) -> ()
  n78 = call <vilib>:"CTRE_Phoenix_MotorControl_RefNumRegistrySet.vi"("refnum name"=w133, "PhoenixMotorControlDevRef"=w92) -> ()  [unwired: 8 in, 2 out]
  n79 = disable-structure shown="Disabled" {
    frame Disabled {
      w175 = "Drive_Motors" ("refnum name")
      n80 = call-poly <vilib>:"WPI_RobotDriveOpen4Motor.vi"() -> ("RobotDriveDevRef"=w177:T32, "error out"=w176:errorcluster)  [unwired: 14 in]
      n81 = call <vilib>:"WPI_RobotDriveRefNum Registry Set.vi"("error in (no error)"=w176, "refnum name"=w175, "RobotDriveDevRef"=w177) -> ("error out"=w178:errorcluster, "RobotDriveDevRef"=w179:T32)  [unwired: 7 in]
      n82 = global write "RefNums_Actuators.vi" "Drive_Motors"(w175) -> ()
      n83 = call <vilib>:"WPI_RobotDriveSafetyConfig.vi"("error in (no error)"=w178, "mode"=WPI_SafetyOutputConfigMenu."Enable", "RobotDriveDevRef"=w179) -> ()  [unwired: 7 in, 2 out]
    }
    frame Enabled {
    }
  }
  n84 = call <vilib>:"CTRE_Phoenix_VictorSPX_Open.vi"("Invert"=FALSE, "Device Number"=u8 23) -> ("CAN Talon SRX Ref"=w78:T27)  [unwired: 8 in, 1 out]
  n85 = call <vilib>:"CTRE_Phoenix_VictorSPX_Open.vi"("Invert"=TRUE, "Device Number"=u8 20) -> ("CAN Talon SRX Ref"=w77:T27)  [unwired: 8 in, 1 out]
  n86 = call <vilib>:"CTRE_Phoenix_VictorSPX_Open.vi"("Invert"=FALSE, "Device Number"=u8 22) -> ("CAN Talon SRX Ref"=w85:T27)  [unwired: 8 in, 1 out]
  n87 = call-poly <vilib>:"WPI_SolenoidOpen.vi"("Reverse Solenoid Channel"=WPI_SolenoidChannel."Solenoid 7", "Forward Solenoid Channel"=WPI_SolenoidChannel."Solenoid 0", "Pneumatics Control Module (0)"=w107) -> ("SolenoidDevRef"=w148:T25)  [unwired: 7 in, 1 out]
  n88 = call-poly <vilib>:"WPI_SolenoidOpen.vi"("Reverse Solenoid Channel"=WPI_SolenoidChannel."Solenoid 6", "Forward Solenoid Channel"=WPI_SolenoidChannel."Solenoid 1", "Pneumatics Control Module (0)"=w107) -> ("SolenoidDevRef"=w117:T25)  [unwired: 7 in, 1 out]
  n89 = call-poly <vilib>:"WPI_SolenoidOpen.vi"("Reverse Solenoid Channel"=WPI_SolenoidChannel."Solenoid 5", "Forward Solenoid Channel"=WPI_SolenoidChannel."Solenoid 2", "Pneumatics Control Module (0)"=w107) -> ("SolenoidDevRef"=w113:T25)  [unwired: 7 in, 1 out]
  n90 = call-poly <vilib>:"WPI_SolenoidOpen.vi"("Reverse Solenoid Channel"=WPI_SolenoidChannel."Solenoid 4", "Forward Solenoid Channel"=WPI_SolenoidChannel."Solenoid 3", "Pneumatics Control Module (0)"=w107) -> ("SolenoidDevRef"=w109:T25)  [unwired: 7 in, 1 out]
  n91 = call <vilib>:"WPI_SolenoidRefNum Registry Set.vi"("refnum name"=w147, "SolenoidDevRef"=w148) -> ()  [unwired: 8 in, 2 out]
  n92 = global write "RefNums_Actuators.vi" "Cargo Arm"(w147) -> ()
  n93 = call <vilib>:"WPI_SolenoidRefNum Registry Set.vi"("refnum name"=w116, "SolenoidDevRef"=w117) -> ()  [unwired: 8 in, 2 out]
  n94 = global write "RefNums_Actuators.vi" "Hatch Arm"(w116) -> ()
  n95 = call <vilib>:"WPI_SolenoidRefNum Registry Set.vi"("refnum name"=w112, "SolenoidDevRef"=w113) -> ()  [unwired: 8 in, 2 out]
  n96 = global write "RefNums_Actuators.vi" "Hatch Eject"(w112) -> ()
  n97 = call <vilib>:"WPI_SolenoidRefNum Registry Set.vi"("refnum name"=w108, "SolenoidDevRef"=w109) -> ()  [unwired: 8 in, 2 out]
  n98 = global write "RefNums_Actuators.vi" "Climber Mantis"(w108) -> ()
  n99 = call <vilib>:"CTRE_Phoenix_MotorControl_ConfigureAllSettings.vi"("timeoutMs"=100, "Motor Controller Configurables"="Victor Enhanced Control", "PhoenixMotorControlDevRef"=w77) -> ("PhoenixMotorControlDevRef"=w80:T27)  [unwired: 7 in, 1 out]
  n100 = call <vilib>:"CTRE_Phoenix_MotorControl_ConfigureAllSettings.vi"("timeoutMs"=100, "Motor Controller Configurables"="Victor Enhanced Control", "PhoenixMotorControlDevRef"=w78) -> ("PhoenixMotorControlDevRef"=w79:T27)  [unwired: 7 in, 1 out]
  n101 = call <vilib>:"CTRE_Phoenix_MotorControl_ConfigureAllSettings.vi"("timeoutMs"=100, "Motor Controller Configurables"="Victor Enhanced Control", "PhoenixMotorControlDevRef"=w85) -> ("PhoenixMotorControlDevRef"=w86:T27)  [unwired: 7 in, 1 out]
  n102 = call <vilib>:"CTRE_Phoenix_MotorControl_SetNeutralMode.vi"("Motor Control Neutral Mode"=CTRE_Phoenix_MotorControl_NeutralMode."Override to Coast", "PhoenixMotorControlDevRef"=w80) -> ("PhoenixMotorControlDevRef"=w81:T27)  [unwired: 8 in, 1 out]
  n103 = call <vilib>:"CTRE_Phoenix_MotorControl_SetNeutralMode.vi"("Motor Control Neutral Mode"=CTRE_Phoenix_MotorControl_NeutralMode."Override to Coast", "PhoenixMotorControlDevRef"=w79) -> ("PhoenixMotorControlDevRef"=w74:T27)  [unwired: 8 in, 1 out]
  n104 = call <vilib>:"CTRE_Phoenix_MotorControl_SetNeutralMode.vi"("Motor Control Neutral Mode"=CTRE_Phoenix_MotorControl_NeutralMode."Override to Coast", "PhoenixMotorControlDevRef"=w86) -> ("PhoenixMotorControlDevRef"=w88:T27)  [unwired: 8 in, 1 out]
  n105 = global write "RefNums_Actuators.vi" "Upper_Intake_PDP"(7 ("Upper_Intake_PDP")) -> ()
  n106 = global write "RefNums_Actuators.vi" "Lower_Intake"(w141) -> ()
  n107 = call <vilib>:"CTRE_Phoenix_MotorControl_RefNumRegistrySet.vi"("refnum name"=w141, "PhoenixMotorControlDevRef"=w81) -> ("PhoenixMotorControlDevRef"=w140:T27)  [unwired: 8 in, 1 out]
  n108 = global write "RefNums_Actuators.vi" "Lower_Intake_PDP"(0 ("Lower_Intake_PDP")) -> ()
  n109 = global write "RefNums_Actuators.vi" "Upper_Intake"(w142) -> ()
  n110 = call <vilib>:"CTRE_Phoenix_MotorControl_RefNumRegistrySet.vi"("refnum name"=w142, "PhoenixMotorControlDevRef"=w74) -> ("PhoenixMotorControlDevRef"=w139:T27)  [unwired: 8 in, 1 out]
  n111 = global write "RefNums_Actuators.vi" "VacuumPump"(w151) -> ()
  n112 = call <vilib>:"CTRE_Phoenix_VictorSPX_Open.vi"("Device Number"=u8 21) -> ("CAN Talon SRX Ref"=w125:T27)  [unwired: 9 in, 1 out]
  n113 = call <vilib>:"WPI_ServoOpen.vi"("Angular Range"=u16 170, "PWM Channel"=FPGA_DIOPWMChannel."PWM 0") -> ("error out"=w37:errorcluster, "ServoDeviceRef"=w34:T33)  [unwired: 8 in]
  n114 = call <vilib>:"CTRE_Phoenix_MotorControl_RefNumRegistrySet.vi"("refnum name"=w151, "PhoenixMotorControlDevRef"=w88) -> ()  [unwired: 8 in, 2 out]
  n115 = global write "RefNums_Actuators.vi" "Spare Victor"(w124) -> ()
  n116 = call <vilib>:"CTRE_Phoenix_MotorControl_RefNumRegistrySet.vi"("refnum name"=w124, "PhoenixMotorControlDevRef"=w125) -> ()  [unwired: 8 in, 2 out]
  n117 = call <vilib>:"WPI_ServoRefNum Registry Set.vi"("error in (no error)"=w37, "refnum name"=w33, "ServoDeviceRef"=w34) -> ()  [unwired: 7 in, 2 out]
  n118 = call <vilib>:"CTRE_Phoenix_MotorControl_ConfigOpenLoopRamp.vi"("secondsFromNeutralToFull"=0.0, "PhoenixMotorControlDevRef"=w140) -> ()  [unwired: 8 in, 2 out]
  n119 = global write "RefNums_Actuators.vi" "Climb Foot Servo"(w33) -> ()
  n120 = call <vilib>:"CTRE_Phoenix_MotorControl_ConfigOpenLoopRamp.vi"("secondsFromNeutralToFull"=0.1, "PhoenixMotorControlDevRef"=w139) -> ()  [unwired: 8 in, 2 out]
  n121 = disable-structure shown="Disabled" {
    disable-tunnel: w132 -> [w181 _]
    frame Disabled {
      n122 = call <vilib>:"WPI_AnalogChannelOpen.vi"("Analog Channel"=FPGA_AIChannel."AI 0") -> ("AIDeviceRef"=w183:T34)  [unwired: 9 in, 1 out]
      n123 = call <vilib>:"WPI_AnalogChannelRefNum Registry Set.vi"("refnum name"=w181, "AIDeviceRef"=w183) -> ()  [unwired: 8 in, 2 out]
    }
    frame Enabled {
    }
  }
  n124 = disable-structure shown="Disabled" {
    disable-tunnel: w131 -> [w184 _]
    frame Disabled {
      n125 = call <vilib>:"WPI_AnalogChannelOpen.vi"("Analog Channel"=FPGA_AIChannel."AI 1") -> ("AIDeviceRef"=w186:T34)  [unwired: 9 in, 1 out]
      n126 = call <vilib>:"WPI_AnalogChannelRefNum Registry Set.vi"("refnum name"=w184, "AIDeviceRef"=w186) -> ()  [unwired: 8 in, 2 out]
    }
    frame Enabled {
    }
  }
  n127 = disable-structure shown="Disabled" {
    disable-tunnel: w130 -> [w187 _]
    frame Disabled {
      n128 = call <vilib>:"WPI_AnalogChannelOpen.vi"("Analog Channel"=FPGA_AIChannel."AI 2") -> ("AIDeviceRef"=w189:T34)  [unwired: 9 in, 1 out]
      n129 = call <vilib>:"WPI_AnalogChannelRefNum Registry Set.vi"("refnum name"=w187, "AIDeviceRef"=w189) -> ()  [unwired: 8 in, 2 out]
    }
    frame Enabled {
    }
  }
  n130 = call-poly <vilib>:"WPI_AccelerometerOpen.vi"("Accel Range"=WPI_AccelerometerRange."+/- 2 g") -> ("error out"=w59:errorcluster, "AccelerometerDevRef"=w60:T35)  [unwired: 9 in]
  n131 = call <vilib>:"WPI_AnalogChannelOpen.vi"("Analog Channel"=FPGA_AIChannel."AI 3") -> ("AIDeviceRef"=w129:T34)  [unwired: 9 in, 1 out]
  n132 = call <vilib>:"WPI_AnalogChannelOpen.vi"("Analog Channel"=FPGA_AIChannel."AI 0") -> ("AIDeviceRef"=w106:T34)  [unwired: 9 in, 1 out]
  n133 = call <vilib>:"WPI_AnalogChannelOpen.vi"("Analog Channel"=FPGA_AIChannel."AI 1") -> ("AIDeviceRef"=w103:T34)  [unwired: 9 in, 1 out]
  n134 = call <vilib>:"WPI_AnalogChannelOpen.vi"("Analog Channel"=FPGA_AIChannel."AI 2") -> ("AIDeviceRef"=w100:T34)  [unwired: 9 in, 1 out]
  n135 = call <vilib>:"WPI_AnalogChannelOpen.vi"("Analog Channel"=FPGA_AIChannel."AI MXP 3") -> ("AIDeviceRef"=w97:T34)  [unwired: 9 in, 1 out]
  n136 = global write "RefNums_Sensors.vi" "Right Prox Sensor"(w132) -> ()
  n137 = call <vilib>:"WPI_AnalogChannelRefNum Registry Set.vi"("refnum name"=w104, "AIDeviceRef"=w106) -> ()  [unwired: 8 in, 2 out]
  n138 = global write "RefNums_Sensors.vi" "Front-Right Prox Sensor"(w104) -> ()
  n139 = call <vilib>:"WPI_AnalogChannelRefNum Registry Set.vi"("refnum name"=w101, "AIDeviceRef"=w103) -> ()  [unwired: 8 in, 2 out]
  n140 = global write "RefNums_Sensors.vi" "Front-Left Prox Sensor"(w101) -> ()
  n141 = call <vilib>:"WPI_AnalogChannelRefNum Registry Set.vi"("refnum name"=w98, "AIDeviceRef"=w100) -> ()  [unwired: 8 in, 2 out]
  n142 = call <vilib>:"WPI_AnalogChannelRefNum Registry Set.vi"("refnum name"=w95, "AIDeviceRef"=w97) -> ()  [unwired: 8 in, 2 out]
  n143 = global write "RefNums_Sensors.vi" "Rear Prox Sensor"(w130) -> ()
  n144 = call <vilib>:"WPI_AnalogChannelRefNum Registry Set.vi"("refnum name"=w127, "AIDeviceRef"=w129) -> ()  [unwired: 8 in, 2 out]
  n145 = global write "RefNums_Sensors.vi" "Upper Pressure Transducer"(w127) -> ()
  n146 = global write "RefNums_Sensors.vi" "Left Prox Sensor"(w131) -> ()
  n147 = global write "RefNums_Sensors.vi" "Tank Pressure Transducer"(w95) -> ()
  n148 = call <vilib>:"WPI_AccelerometerRefNum Registry Set.vi"("error in (no error)"=w59, "refnum name"=w57, "AccelerometerDevRef"=w60) -> ()  [unwired: 7 in, 2 out]
  n149 = global write "RefNums_Sensors.vi" "Ground Prox Sensor"(w98) -> ()
  n150 = global write "RefNums_Sensors.vi" "Accelerometer"(w57) -> ()
  "error out" <- "error in"
